vi "Refresh External.vi"(8 "error in (no error)":errorcluster, 11 "BluelinesRedlines in":refnum<class "BluelinesRedlines.lvclass">) -> (0 "error out":errorcluster, 3 "BluelinesRedlines out":refnum<class "BluelinesRedlines.lvclass">)   [LabVIEW 2020, in "VolatusGUIElements.lvlib" / "BluelinesRedlines.lvclass"]
uses:
  BluelinesRedlines.lvclass
  BluelinesRedlines.lvclass/BluelinesRedlines.ctl
  VolatusGUI/BluelinesRedlines Source/BluelinesRedlines Source.lvclass
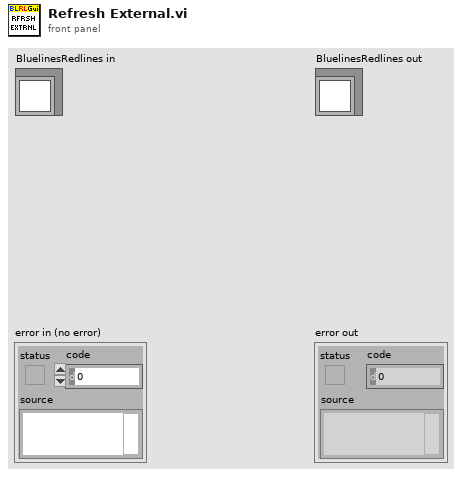
[diagram p1: front panel]
types:
  T1 = map{string, refnum<class "BluelinesRedlines Source.lvclass">}
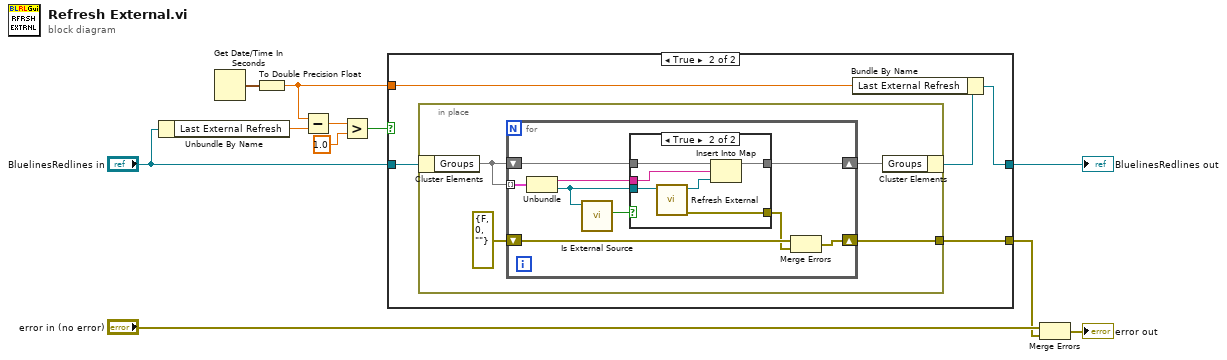
[diagram p0: block diagram]
diagram:
  n1 = Unbundle By Name("BluelinesRedlines in") -> ("Last External Refresh"=w6:dbl)
  n2 = Get Date/Time In Seconds() -> (seconds since 1Jan1904=w7:timestamp)
  n3 = To Double Precision Float(number=w7) -> (double precision float=w2:dbl)
  n4 = Subtract(x=w2, y=w6) -> (x-y=w5:dbl)
  n5 = Greater?(x=w5, y=1.0) -> (0:w3:bool)
  n6 = case shown="True" w3 {
    tunnel: [_ w16] -> w9
    tunnel: "BluelinesRedlines in" -> [w12 w15]
    tunnel: w2 -> [_ w13]
    tunnel: [w12 w14] -> w1
    frame False {
    }
    frame True {
      n7 = in-place {
        in-place-border: [w18] -> w16
        n8 = in-place-cluster #1(w15) -> ("Groups"=w21:T1)
        n9 = for {
          shift-right: [w25] -> w20
          shift-left: w21 -> [w26]
          tunnel: w21 -> [w30] mode=indexing
          shift-right: [w22] -> w18
          shift-left: errorcluster {"status"=FALSE, "code"=0, "source"=""} ("error constant") -> [w24]
          n10 = Unbundle(w30) -> ("Name"=w27:string, "VolatusGUI:BluelinesRedlines Source.lvclass"=w28:refnum<class "BluelinesRedlines Source.lvclass">)
          n11 = call-dynamic "Is External Source.vi"("BluelinesRedlines Source in"=w28) -> ("External Source"=w29:bool)  [unwired: 10 in]
          n12 = case shown="True" w29 {
            tunnel: w28 -> [_ w37]
            tunnel: w27 -> [_ w34]
            tunnel: w26 -> [w31 w36]
            tunnel: [w31 w33] -> w25
            tunnel: [_ w32] -> w23
            frame False {
            }
            frame True {
              n13 = call-dynamic "Refresh External.vi"("BluelinesRedlines Source in"=w37) -> ("error out"=w32:errorcluster, "BluelinesRedlines Source out"=w35:refnum<class "BluelinesRedlines Source.lvclass">)  [unwired: 9 in]
              n14 = Insert Into Map(map in=w36, key=w34, value=w35) -> (map out=w33:T1)  [unwired: 2 out]
            }
          }
          n15 = Merge Errors(w24, w23) -> (w22:errorcluster)
        }
        n16 = in-place-cluster #1("Groups"=w20) -> (w17:refnum<class "BluelinesRedlines.lvclass">)
      }
      n17 = Bundle By Name(cluster=w17, "Last External Refresh"=w13) -> (w14:refnum<class "BluelinesRedlines.lvclass">)
    }
  }
  "BluelinesRedlines out" <- w1
  n18 = Merge Errors("error in (no error)", w9) -> (→"error out":errorcluster)
